vi "RelayAndCompressor.vi"() -> ()   [LabVIEW 2013]
doc: "This example shows how to control a relay.\n\nThis example works with the NI 9403 module connected to a Digital Sidecar. The Digital Sidecar should have 12V applied to the WAGO connector. This example uses a standard PWM cable with the female end connected to the Digital Sidecar and the male end connected to the 3-pin terminal on the SPIKE relay. The white wire of the PWM cable connects from the <B>A</B> relay output to the left socket of the SPIKE 3-pin terminal. The red PWM wire connects between the <B>B</B> relay output and the center socket of the SPIKE 3-pin terminal. The black PWM wire connects between the <B>(-)</B> relay terminal and the <B>B</B> socket of the SPIKE 3-pin terminal."
uses:
  <vilib>/Rock Robotics/WPI/Relay/WPI_RelayValue.ctl
  <vilib>/Rock Robotics/WPI/Relay/WPI_RelayDirection.ctl
  <vilib>/Rock Robotics/SystemInterfaces/DIO/FPGA_DIORelayChannel.ctl
  <vilib>/Rock Robotics/SystemInterfaces/Typedef/FPGA_TypedefDigitalModule.ctl
  <vilib>/Rock Robotics/SystemInterfaces/DIO/FPGA_DIOChannel.ctl
panel:
  out "for/rev":bool
  out "on/off":bool
  in  "stop":bool
  in  "RelayValue":T1
  # "Wiring Diagram for Digital Sidecar connected to an NI 9403"
  # "Set these inputs before running."
  # "This can be set while running."
  # "(-)"
  # "B"
  # "A"
  # "8\n7\n6\n5\n4\n3\n2\n1"
  # "RELAY"
  # "Connect\nPower\nHere"
  # "GND"
  # "M-"
  # "Connect\nLoad\nHere"
  # "Off = Amber\nOn = ---\nForward = Green\nReverse = Red"
  # "SPIKE"
  # "12V"
  # "M+"
  # "B"
  # "20A"
  # "fuse"
  # "PWM cable"
  # "Digital Sidecar"
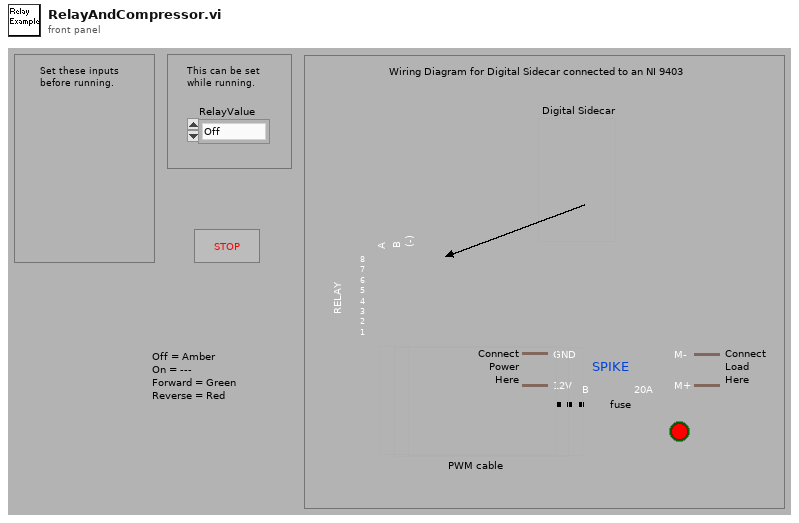
[diagram p1: front panel]
types:
  T1 = typedef "WPI_RelayValue.ctl" = enum16{"Off", "On", "Forward", "Reverse"}
  T2 = typedef "FPGA_TypedefDigitalModule.ctl" = enum16{"Digital Module 1", "Digital Module 2"}
  T3 = typedef "FPGA_DIORelayChannel.ctl" = enum8{"Relay 1", "Relay 2", "Relay 3", "Relay 4", "Relay 5", "Relay 6", "Relay 7", "Relay 8", "Invalid"}
  T4 = typedef "WPI_RelayDirection.ctl" = enum16{"Both directions", "Forward only", "Reverse only"}
  T5 = typedef "FPGA_DIOChannel.ctl" = enum8{"DIO 1", "DIO 2", "DIO 3", "DIO 4", "DIO 5", "DIO 6", "DIO 7", "DIO 8", "DIO 9", "DIO 10", "DIO 11", "DIO 12", "DIO 13", "DIO 14", "Invalid"}
  T6 = typedef "WPI_CompressorDevRef.ctl" = cluster{"DevStatus":errorcluster, "DigitalInputDevRef":T7, "RelayDevRef":T8}
  T7 = typedef "WPI_DigitalInputDevRef.ctl" = cluster{"DevStatus":errorcluster, "DIO Channel":T5, "Digital Module":T2}
  T8 = typedef "WPI_RelayDevRef.ctl" = cluster{"DevStatus":errorcluster, "Relay Channel":T3, "Digital Module":T2, "Relay Direction":T4}
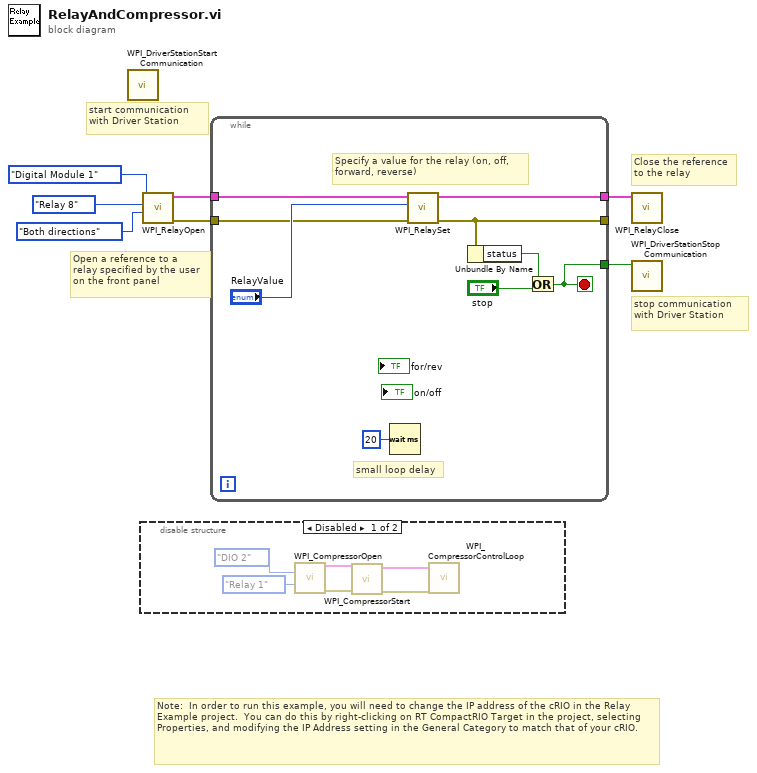
[diagram p0: block diagram]
diagram:
  # "stop communication with Driver Station"
  # "start communication with Driver Station"
  # "Note:  In order to run this example, you will need to change the IP address of the cRIO in the Relay Example project.  You can do this by right-clicking on RT CompactRIO Target in the project, selecting Properties, and modifying the IP Address setting in the General Category to match that of your cRIO."
  # "Close the reference\nto the relay"
  # "Open a reference to a \nrelay specified by the user\non the front panel"
  n1 = call <vilib>:"WPI_DriverStationStart Communication.vi"() -> ()  [unwired: 1 in, 11 out]
  n2 = disable-structure shown="Disabled" {
    frame Disabled {
      n3 = call <vilib>:"WPI_CompressorOpen.vi"("Pressure Switch DIO Channel"=FPGA_DIOChannel."DIO 2", "Relay Channel"=FPGA_DIORelayChannel."Relay 1") -> ("CompressorDevRef"=w10:T6, "error out"=w11:errorcluster)  [unwired: 12 in]
      n4 = call <vilib>:"WPI_CompressorStart.vi"("error in (no error)"=w11, "CompressorDevRef"=w10) -> ("error out"=w8:errorcluster, "CompressorDevRef"=w9:T6)  [unwired: 8 in]
      n5 = call <vilib>:"WPI_CompressorControlLoop.vi"("error in (no error)"=w8, "CompressorDevRef"=w9) -> ()  [unwired: 10 in]
    }
    frame Enabled {
    }
  }
  n6 = call <vilib>:"WPI_RelayOpen.vi"("Relay Direction"=WPI_RelayDirection."Both directions" ("RelayDirection"), "Relay Channel"=FPGA_DIORelayChannel."Relay 8" ("RelayChannel"), "Digital Module (Module 1)"=FPGA_TypedefDigitalModule."Digital Module 1" ("DIO Module")) -> ("error out"=w1:errorcluster, "RelayDevRef"=w7:T8)  [unwired: 1 in, 6 out]
  n7 = while {
    tunnel: w7 -> [w22]
    tunnel: [w21] -> w6
    tunnel: [w16] -> w4
    tunnel: w1 -> [w15]
    tunnel: [w14] -> _
    stop <- w16 stop-if-true
    # "small loop delay"
    # "Specify a value for the relay (on, off, \nforward, reverse)"
    n8 = Wait (ms)(milliseconds to wait=u32 20) -> ()  [unwired: 1 out]
    n9 = call <vilib>:"WPI_RelaySet.vi"("error in (no error)"=w15, "RelayValue"="RelayValue", "RelayDevRef"=w22) -> ("error out"=w14:errorcluster, "RelayDevRef"=w21:T8)  [unwired: 7 out]
    n10 = Unbundle By Name(w14) -> ("status"=w17:bool)
    n11 = Or(x=w17, y="stop") -> (x .or. y?=w16:bool)
  }
  n12 = call <vilib>:"WPI_RelayClose.vi"("RelayDevRef"=w6) -> ()  [unwired: 1 in, 10 out]
  n13 = call <vilib>:"WPI_DriverStationStop Communication.vi"("StopCommunication"=w4) -> ()  [unwired: 1 in, 10 out]
